vi "Read Msg Input.vi"(10 "Msg Input":refnum<class "Msg Input.lvclass">) -> (4 "Teller":refnum<class "Teller.lvclass">)   [LabVIEW 2020, in "_Template.lvlib" / "Templates.lvlib" / "TEMPLATE jettl Msg.lvlib" / "TEMPLATE Msg Input.lvlib"]
uses:
  TEMPLATE Msg Input.lvlib
  jettl/jettl/Teller/Teller.lvclass
  jettl/jettl/Msg Input/Msg Input.lvclass
  TEMPLATE Msg Input/TEMPLATE Msg Input.lvclass
panel:
  # "This front panel should not be manipulated."
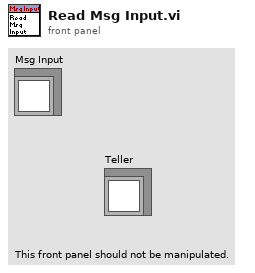
[diagram p1: front panel]
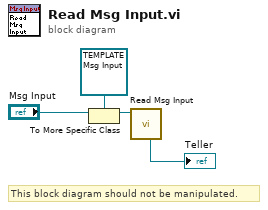
[diagram p0: block diagram]
diagram:
  # "This block diagram should not be manipulated."
  n1 = To More Specific Class(target class=refnum<class "TEMPLATE Msg Input.lvclass"> refnum ("_Template.lvlib:Templates.lvlib:TEMPLATE Msg.lvlib:TEMPLATE Msg Input.lvlib:TEMPLATE Msg Input.lvclass"), reference="Msg Input") -> (specific class reference=w2:refnum<class "TEMPLATE Msg Input.lvclass">)  [unwired: 1 in, 1 out]
  n2 = call "Read Msg Input.vi"("TEMPLATE Msg Input in"=w2) -> ("Teller"=→"Teller":refnum<class "Teller.lvclass">)  [unwired: 10 in]
